vi "MDAQ_Settings_Set.vi"(8 "error in":errorcluster, 9 "Status_Cluster":T1 {"GATESTOP" format="%04x"; "GATESTRT" format="%04x"; "AMPLITUDE" format="%04x"; "M_CYCLES" format="%04x"; "N_CYCLES" format="%04x"; "STEP" format="%04x"; "BASE" format="%04x"; "CHAN" format="%04x"}, 10 "ARG Cluster":T2, 11 "VISA resource name":refnum<visa-resource-name>) -> (0 "error out":errorcluster, 1 "Status_Cluster Out":T1 {"GATESTOP" format="%04x"; "GATESTRT" format="%04x"; "AMPLITUDE" format="%04x"; "M_CYCLES" format="%04x"; "N_CYCLES" format="%04x"; "STEP" format="%04x"; "BASE" format="%04x"; "CHAN" format="%04x"}, 3 "VISA resource name out":refnum<visa-resource-name>)   [LabVIEW 2021]
uses:
  Status_Cluster.ctl
  ARG_Cluster.ctl
  CMD_ARG_Enum.ctl
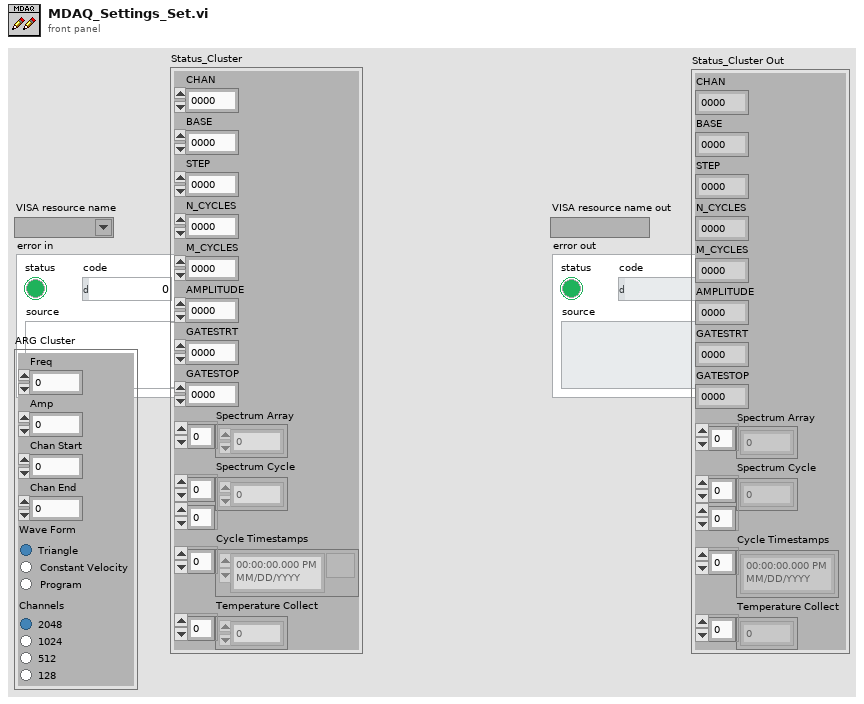
[diagram p1: front panel]
types:
  T1 = typedef "Status_Cluster.ctl" = cluster{"CHAN":u32, "BASE":u32, "STEP":u32, "N_CYCLES":u32, "M_CYCLES":u32, "AMPLITUDE":u32, "GATESTRT":u32, "GATESTOP":u32, "Spectrum Array":u32[], "Spectrum Cycle":u32[][], "Cycle Timestamps":timestamp[], "Temperature Collect":dbl[]}
  T2 = typedef "ARG_Cluster.ctl" = cluster{"Freq":dbl, "Amp":dbl, "Chan Start":dbl, "Chan End":dbl, "Wave Form":enum32{"Item 0", "Item 1", "Radio Selection 3"}, "Channels":enum32{"Item 0", "Item 1", "Radio Selection 3", ""}}
  T3 = typedef "CMD_ARG_Enum.ctl" = enum16{"N_Cycles", "GateStep", "ASCII_Spectrum", "Waveform", "GateStop", "GateStart", "Amplitude", "Frequency"}
  T4 = enum32{"Item 0", "Item 1", "Radio Selection 3", ""}
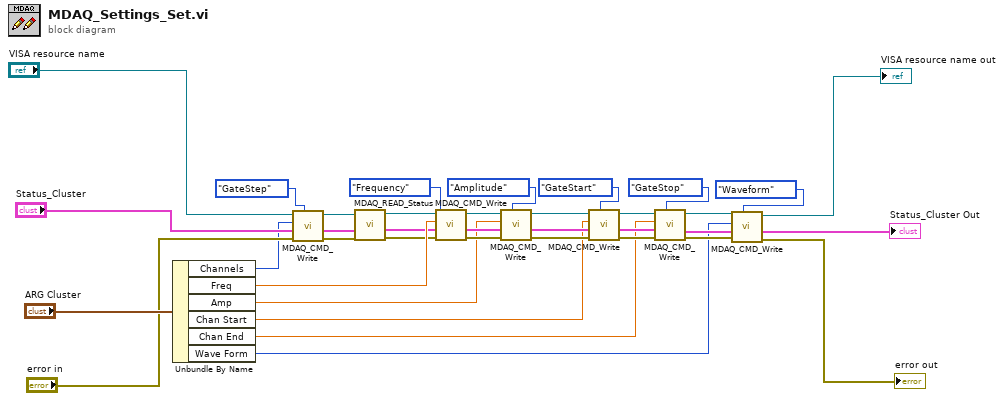
[diagram p0: block diagram]
diagram:
  n1 = Unbundle By Name("ARG Cluster") -> ("Channels"=w1:T4, "Freq"=w36:dbl, "Amp"=w31:dbl, "Chan Start"=w26:dbl, "Chan End"=w21:dbl, "Wave Form"=w16:enum32{"Item 0", "Item 1", "Radio Selection 3"})
  n2 = call "MDAQ_CMD_Write.vi"("CMD"=CMD_ARG_Enum."GateStep", "error in"="error in", "Status_Cluster"="Status_Cluster", "ARG"=w1, "VISA resource name"="VISA resource name") -> ("error out"=w7:errorcluster, "Status_Cluster Out"=w6:T1, "VISA resource name out"=w8:refnum<visa-resource-name>)  [unwired: 4 in]
  n3 = call "MDAQ_READ_Status.vi"("error in"=w7, "Status_Cluster IN"=w6, "VISA resource name"=w8) -> ("error out"=w10:errorcluster, "output cluster"=w9:T1, "VISA resource name out"=w11:refnum<visa-resource-name>)  [unwired: 6 in]
  n4 = call "MDAQ_CMD_Write.vi"("CMD"=CMD_ARG_Enum."Frequency", "error in"=w10, "Status_Cluster"=w9, "ARG"=w36, "VISA resource name"=w11) -> ("error out"=w33:errorcluster, "Status_Cluster Out"=w32:T1, "VISA resource name out"=w34:refnum<visa-resource-name>)  [unwired: 4 in]
  n5 = call "MDAQ_CMD_Write.vi"("CMD"=CMD_ARG_Enum."Amplitude", "error in"=w33, "Status_Cluster"=w32, "ARG"=w31, "VISA resource name"=w34) -> ("error out"=w28:errorcluster, "Status_Cluster Out"=w27:T1, "VISA resource name out"=w29:refnum<visa-resource-name>)  [unwired: 4 in]
  n6 = call "MDAQ_CMD_Write.vi"("CMD"=CMD_ARG_Enum."GateStart", "error in"=w28, "Status_Cluster"=w27, "ARG"=w26, "VISA resource name"=w29) -> ("error out"=w23:errorcluster, "Status_Cluster Out"=w22:T1, "VISA resource name out"=w24:refnum<visa-resource-name>)  [unwired: 4 in]
  n7 = call "MDAQ_CMD_Write.vi"("CMD"=CMD_ARG_Enum."GateStop", "error in"=w23, "Status_Cluster"=w22, "ARG"=w21, "VISA resource name"=w24) -> ("error out"=w18:errorcluster, "Status_Cluster Out"=w17:T1, "VISA resource name out"=w19:refnum<visa-resource-name>)  [unwired: 4 in]
  n8 = call "MDAQ_CMD_Write.vi"("CMD"=CMD_ARG_Enum."Waveform", "error in"=w18, "Status_Cluster"=w17, "ARG"=w16, "VISA resource name"=w19) -> ("error out"=→"error out":errorcluster, "Status_Cluster Out"=→"Status_Cluster Out":T1, "VISA resource name out"=→"VISA resource name out":refnum<visa-resource-name>)  [unwired: 4 in]
